vi "Read Publisher Instance.vi"(8 "error in":errorcluster, 11 "CoreOOB_Rx in":refnum<class "CIFCoreOOB_Rx.lvclass">) -> (0 "error out":errorcluster, 2 "Publisher Instance":T1, 3 "CoreOOB_Rx out":refnum<class "CIFCoreOOB_Rx.lvclass">)   [LabVIEW 2021, in "CIFCoreOOB_Rx.lvclass"]
uses:
  CIFCoreOOB_Rx.lvclass
  C:/Program Files/National Instruments/LabVIEW 2021/vi.lib/CIF Foundation/CIF Out of Band Commands/CIFOutOfBand.lvclass
  <vilib>/CIF Foundation/CIF Out of Band Commands/CIFOutOfBand.lvclass/CIFOutOfBand.ctl
  <vilib>/CIF Foundation/CIF Out of Band Commands/Accessors/Read Local OOB Data.vi
  CIFCoreOOB_Rx.lvclass/CIFCoreOOB_Rx.ctl
  <vilib>/CIF Foundation/CIF Channels Core/ChannelCommon/typedef/New FIFO Instance Configuration.ctl
  <vilib>/CIF Foundation/CIF Channels Core/ChannelCommon/ChannelCommon.lvlib
  Typedef/FIFO Publisher.ctl
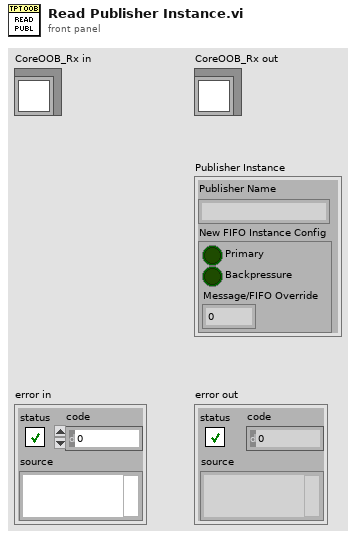
[diagram p1: front panel]
types:
  T1 = typedef "CIFCoreOOB_Rx.lvclass/FIFO Publisher.ctl" = cluster{"Publisher Name":string, "New FIFO Instance Config":T2}
  T2 = typedef "ChannelCommon.lvlib/New FIFO Instance Configuration.ctl" = cluster{"Primary":bool, "Backpressure":bool, "Message/FIFO Override":u32}
  T3 = typedef "CIFCoreOOB_Rx.lvclass/Template Payload.ctl" = cluster{"Config Data":variant, "Clock Conversion":T4, "Connections":T6[], "Forces":T7[], "Publisher Instance":T1}
  T4 = typedef "Time_CIF_U.lvlib/Clock Conversion Map.ctl" = map{u8, cluster{"Last Reset":i64, "Offset Pair":T5, "Slope":dbl, "1/Slope":dbl}}
  T5 = typedef "Time_CIF_U.lvlib/Timestamp Pair.ctl" = cluster{"System Time":i64, "External Time":i64}
  T6 = typedef "CIFCoreOOB_Rx.lvclass/Channel Connection Data.ctl" = cluster{"Publisher Name":string, "Subscriber Name":string, "Connection Data":u8[]}
  T7 = typedef "CIFCoreOOB_Rx.lvclass/Channel Fault Data.ctl" = cluster{"Channel Name":string, "Force Data":u8[], "Force Active":bool}
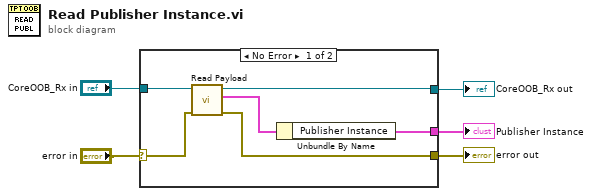
[diagram p0: block diagram]
diagram:
  n1 = case shown="No Error" "error in" {
    selector: "error in" -> [w11 w13]
    tunnel: [w9 w13] -> w5
    tunnel: [w6 w12] -> w4
    tunnel: "CoreOOB_Rx in" -> [w8 w12]
    tunnel: [w7 _] -> w1
    frame No Error {
      n2 = call "Read Payload.vi"("error in"=w11, "CoreOOB_Rx in"=w8) -> ("error out"=w9:errorcluster, "data"=w10:T3, "CoreOOB_Rx out"=w6:refnum<class "CIFCoreOOB_Rx.lvclass">)  [unwired: 7 in]
      n3 = Unbundle By Name(w10) -> ("Publisher Instance"=w7:T1)
    }
    frame Error {
    }
  }
  "error out" <- w5
  "CoreOOB_Rx out" <- w4
  "Publisher Instance" <- w1
